vi "Untitled 6.vi"() -> ()   [LabVIEW 2019]
uses:
  Generated_client/RPC Messages/Greeter_req.ctl
  Generated_client/RPC Messages/Greeter_req_req_oneof/Greeter_req_req_oneof.lvclass
  Generated_client/RPC Messages/Greeter_req_req_oneof/Greeter_req_req_oneof.lvclass/Greeter_req_req_oneof.ctl
  Generated_client/RPC Messages/Greeter_res_res_oneof/Greeter_res_res_oneof.lvclass/Greeter_res_res_oneof.ctl
  Generated_client/Generated_client.lvlib
  Generated_client/RPC Messages/Greeter_res_res_oneof/Greeter_res_res_oneof.lvclass
panel:
  out "Has Data? 2":bool
  out "Has Data?":bool
  out "Get_Val":i32
  out "res_latitude":i32
  in  "Set_Val":i32
  in  "Request Data":T1
  out "error out":errorcluster
  in  "address":string
  in  "error in":errorcluster
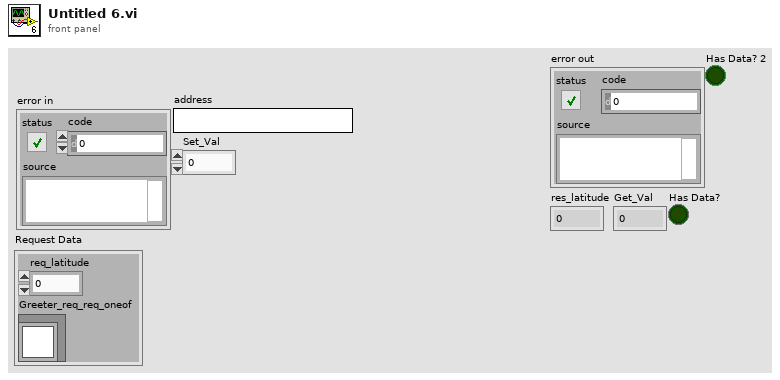
[diagram p1: front panel]
types:
  T1 = typedef "Generated_client.lvlib/Greeter_req.ctl" = cluster{"req_latitude":i32, "Greeter_req_req_oneof":refnum<class "Greeter_req_req_oneof.lvclass">}
  T2 = typedef "grpc-lvsupport-release.lvlib/grpcId.ctl" = u64
  T3 = typedef "Generated_client.lvlib/Greeter_res.ctl" = cluster{"res_latitude":i32, "Greeter_res_res_oneof":refnum<class "Greeter_res_res_oneof.lvclass">}
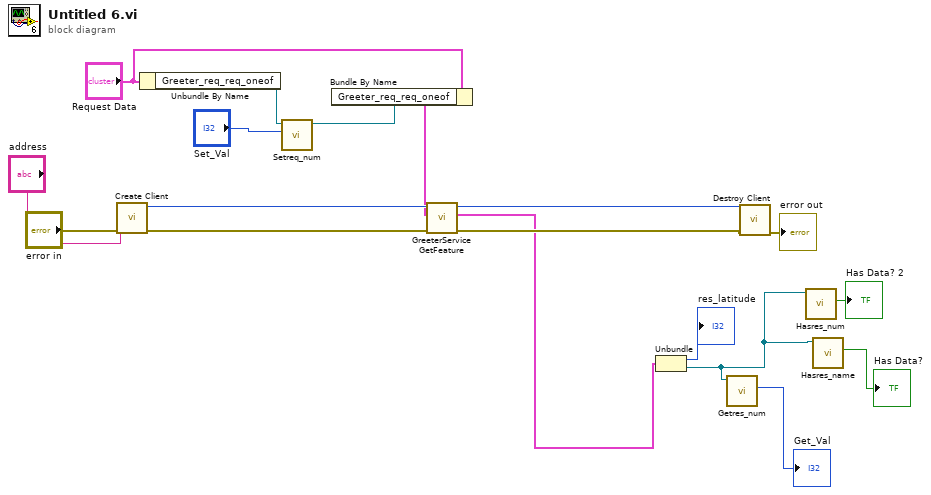
[diagram p0: block diagram]
diagram:
  n1 = call "Create Client.vi"("error in"="error in", "address"="address") -> ("error out"=w16:errorcluster, "gRPC ID Out"=w18:T2)  [unwired: 8 in]
  n2 = Unbundle By Name("Request Data") -> ("Greeter_req_req_oneof"=w8:refnum<class "Greeter_req_req_oneof.lvclass">)
  n3 = call "Setreq_num.vi"("Set_Val"="Set_Val", "OneOfTemplate in"=w8) -> ("OneOfTemplate out"=w7:refnum<class "Greeter_req_req_oneof.lvclass">)  [unwired: 8 in, 1 out]
  n4 = Bundle By Name(cluster="Request Data", "Greeter_req_req_oneof"=w7) -> (w10:T1)
  n5 = call "GreeterService GetFeature.vi"("error in"=w16, "Request Data"=w10, "gRPC ID"=w18) -> ("error out"=w15:errorcluster, "Response Data"=w9:T3, "gRPC ID out"=w17:T2)  [unwired: 6 in]
  n6 = Unbundle(w9) -> ("res_latitude"=→"res_latitude":i32, "Greeter_res_res_oneof"=w4:refnum<class "Greeter_res_res_oneof.lvclass">)
  n7 = call "Getres_num.vi"("OneOfTemplate in"=w4) -> ("Get_Val"=→"Get_Val":i32)  [unwired: 8 in, 2 out]
  n8 = call "Destroy Client.vi"("error in"=w15, "gRPC ID"=w17) -> ("error out"=→"error out":errorcluster)  [unwired: 9 in]
  n9 = call "Hasres_num.vi"("OneOfTemplate in"=w4) -> ("Has Data?"=→"Has Data? 2":bool)  [unwired: 8 in, 2 out]
  n10 = call "Hasres_name.vi"("OneOfTemplate in"=w4) -> ("Has Data?"=→"Has Data?":bool)  [unwired: 8 in, 2 out]
